vi "Serial Calc Timing Values.vi"(6 "FPGA Clock Rate (40000000)":u32=40000000, 7 "baud rate (1000000)":u32=1000000) -> (0 "Two Bit":u32, 1 "One and Half Bit":u32, 2 "One Bit":u32, 3 "Half Bit":u32)   [LabVIEW 2016]
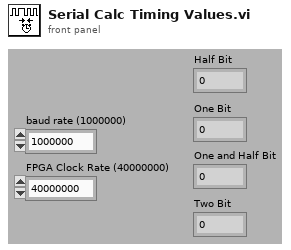
[diagram p1: front panel]
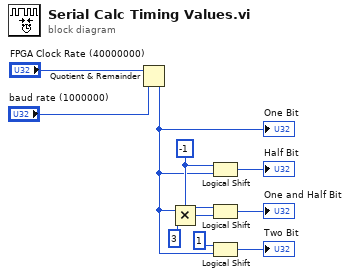
[diagram p0: block diagram]
diagram:
  w8 = i16 -1 ("y")
  n1 = Quotient & Remainder(x="FPGA Clock Rate (40000000)", y="baud rate (1000000)") -> (floor(x/y)=w4:u32)  [unwired: 1 out]
  "One Bit" <- w4
  n2 = Multiply(x=w4, y=u32 3) -> (x*y=w10:u32)
  n3 = Logical Shift(y=w8, x=w4) -> (x << y=→"Half Bit":u32)
  n4 = Logical Shift(y=w8, x=w10) -> (x << y=→"One and Half Bit":u32)
  n5 = Logical Shift(y=i16 1, x=w4) -> (x << y=→"Two Bit":u32)
